vi "Write Tracker Msg.vi"(5 "Action(Start)":T1, 6 "Message Priority(Normal)":T2=enum."Normal", 7 "Publish Data?(T)":bool=TRUE, 8 "error in (no error)":errorcluster, 9 "Timeout if Waiting(-1ms)":i32=-1, 10 "Send Function(Await Reply)":T3=enum."Await Reply", 11 "Data Tracker Msg in":refnum<class "Data Tracker Msg.lvclass">) -> (0 "error out":errorcluster, 3 "Data Tracker Msg out":refnum<class "Data Tracker Msg.lvclass">)   [LabVIEW 2020, in "Data Tracker.lvlib" / "Data Tracker Msg.lvclass"]
doc: "Write the private data of the Data Tracker Msg."
uses:
  Data Tracker Msg.lvclass
  PPL/HDH.Actor Framework.Core.Publisher.lvlibp/Messages/Response Msg/Response Core/Controls/Ctl_SendFunction.ctl
  PPL/HDH.Actor Framework.Core.Actor.lvlibp/1abvi3w/vi.lib/ActorFramework/Message Enqueuer/Message Priority.ctl
  Controls/Ctl_Action.ctl
  Data Tracker Msg.lvclass/Data Tracker Msg.ctl
  PPL/HDH.Actor Framework.Core.Publisher.lvlibp
  PPL/HDH.Actor Framework.Core.Actor.lvlibp/1abvi3w/vi.lib/ActorFramework/Message Enqueuer/Message Enqueuer.lvclass
  Data Tracker.lvlib
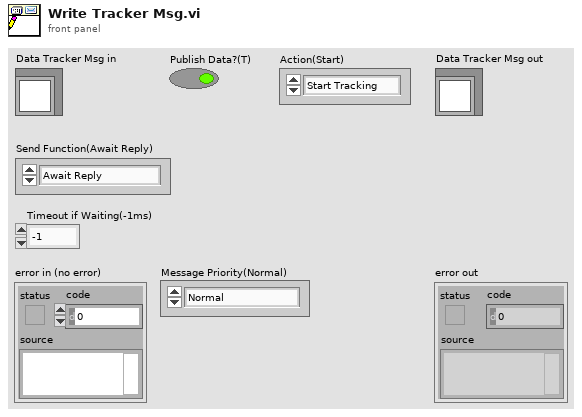
[diagram p1: front panel]
types:
  T1 = typedef "Data Tracker.lvlib/Ctl_Action.ctl" = enum16{"Start Tracking", "End Tracking", "Abort Tracking"}
  T2 = typedef "HDH.Actor Framework.Core.Actor.lvlibp/Message Enqueuer.lvclass/Message Priority.ctl" = enum16{"Low", "Normal", "High"}
  T3 = typedef "HDH.Actor Framework.Core.Publisher.lvlibp/Ctl_SendFunction.ctl" = enum16{"Send and Forget", "Request Reply", "Await Reply"}
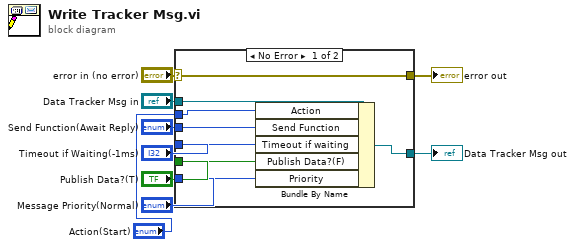
[diagram p0: block diagram]
diagram:
  n1 = case shown="No Error" "error in (no error)" {
    selector: "error in (no error)" -> [w17 w18]
    tunnel: [w17 w18] -> w8
    tunnel: [w15 w19] -> w6
    tunnel: "Data Tracker Msg in" -> [w16 w19]
    tunnel: "Send Function(Await Reply)" -> [w12 _]
    tunnel: "Publish Data?(T)" -> [w11 _]
    tunnel: "Timeout if Waiting(-1ms)" -> [w14 _]
    tunnel: "Message Priority(Normal)" -> [w13 _]
    tunnel: "Action(Start)" -> [w10 _]
    frame No Error {
      n2 = Bundle By Name(cluster=w16, "Action"=w10, "Send Function"=w12, "Timeout if waiting"=w14, "Publish Data?(F)"=w11, "Priority"=w13) -> (w15:refnum<class "Data Tracker Msg.lvclass">)
    }
    frame Error {
    }
  }
  "error out" <- w8
  "Data Tracker Msg out" <- w6
